vi "Init TSF.vi"(8 "error in (no error)":errorcluster, 11 "QPA Measurement in":refnum<class "QPA Measurement.lvclass">) -> (0 "error out":errorcluster, 3 "QPA Measurement out":refnum<class "QPA Measurement.lvclass">)   [LabVIEW 2016, in "QPA Measurement.lvlib" / "QPA Measurement.lvclass"]
uses:
  QPA Measurement.lvclass
  C:/Projects/STS/Common/Sequence Automation/Plugins/Measurement Interface.lvlibp/Measurement Interface.lvclass
  Plugins/TSF Parser.lvlibp/TSF Parser.lvclass
  QPA Measurement.lvclass/QPA Measurement.ctl
  Plugins/Measurement Interface.lvlibp/Private Methods/Active Sequence File/Read Active Sequence File.vi
  Plugins/TestStand API Tools (TSAT).lvlibp/Sequence File Actions/TSAT Sequence File Actions.lvlib
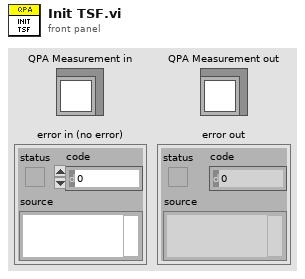
[diagram p1: front panel]
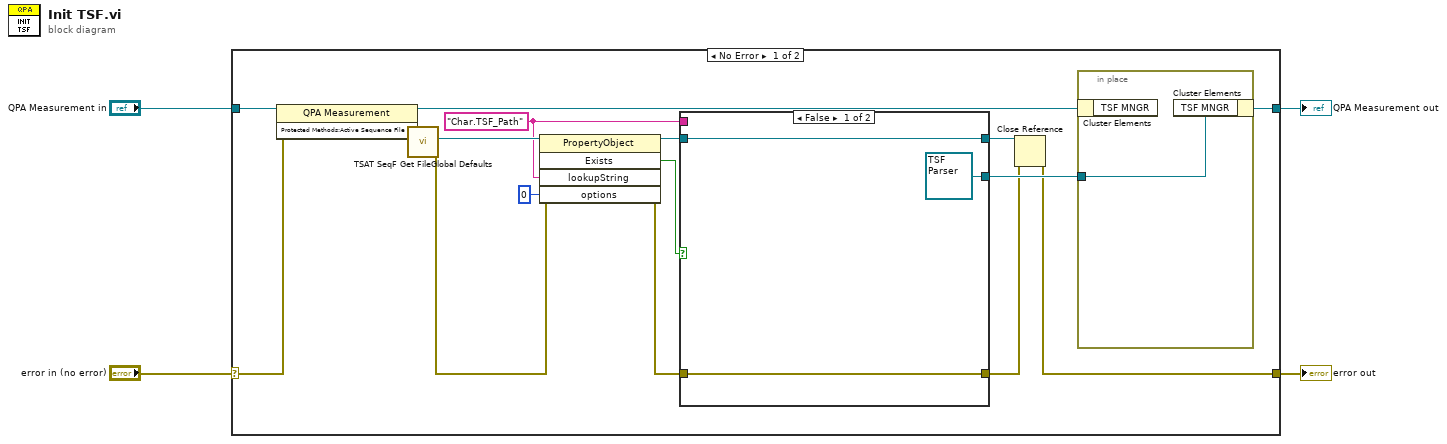
[diagram p0: block diagram]
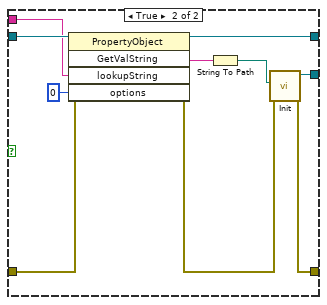
[diagram p2: hidden frame]
diagram:
  n1 = case shown="No Error" "error in (no error)" {
    selector: "error in (no error)" -> [w21 w37]
    tunnel: [w6 w37] -> w3
    tunnel: [w19 w36] -> w1
    tunnel: "QPA Measurement in" -> [w18 w36]
    frame No Error {
      w10 = "Char.TSF_Path" ("lookupString")
      n2 = property class="QPA Measurement"(reference=w18, error in=w21) -> (reference out=w17:refnum<class "QPA Measurement.lvclass">, error out=w15:errorcluster, "Protected Methods:Active Sequence File"=w16:refnum<k7>)
      n3 = call "TSAT SeqF Get FileGlobal Defaults.vi"("Error In"=w15, "Sequence File In"=w16) -> ("Error Out"=w14:errorcluster, "FileGlobalsDefaultValues"=w12:refnum<k7>)  [unwired: 7 in, 1 out]
      n4 = invoke class="PropertyObject" method="Exists"(reference=w12, error in=w14, "lookupString"=w10, "options"=0) -> (reference out=w11:refnum<k7>, error out=w13:errorcluster, "Exists"=w9:bool)  [unwired: 1 in, 2 out]
      n5 = case shown="False" w9 {
        tunnel: [w24 w34] -> w5
        tunnel: [refnum<class "TSF Parser.lvclass"> refnum ("TSF Parser out") w33] -> w20
        tunnel: w13 -> [w24 w31]
        tunnel: w11 -> [w22 w30]
        tunnel: w10 -> [_ w29]
        tunnel: [w22 w25] -> w7
        frame False {
        }
        frame True {
          n6 = invoke class="PropertyObject" method="GetValString"(reference=w30, error in=w31, "lookupString"=w29, "options"=0) -> (reference out=w25:refnum<k7>, error out=w32:errorcluster, "GetValString"=w27:string)  [unwired: 1 in, 2 out]
          n7 = String To Path(string=w27) -> (path=w26:path)
          n8 = call "Init.vi"("error in (no error)"=w32, "TSF File Path"=w26) -> ("error out"=w34:errorcluster, "TSF Parser out"=w33:refnum<class "TSF Parser.lvclass">)  [unwired: 8 in]
        }
      }
      n9 = Close Reference(reference=w7, error in (no error)=w5) -> (error out=w6:errorcluster)
      n10 = in-place {
        in-place-border: w20 -> [w35]
        n11 = in-place-cluster #1(w17) -> ()  [unwired: 1 out]
        n12 = in-place-cluster #1("TSF MNGR"=w35) -> (w19:refnum<class "QPA Measurement.lvclass">)
      }
    }
    frame Error {
    }
  }
  "error out" <- w3
  "QPA Measurement out" <- w1
